vi "CarSimulator.vi"(10 "Steering Control":dbl, 11 "Brake/Gas Control":dbl) -> (1 "Acceleration":dbl, 2 "Velocity":dbl, 3 "Position":dbl)   [LabVIEW 2020]
panel:
  in  "Gas to Acceleration Scalar":dbl=1.8
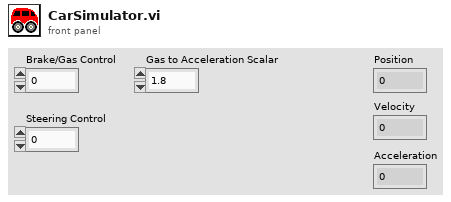
[diagram p1: front panel]
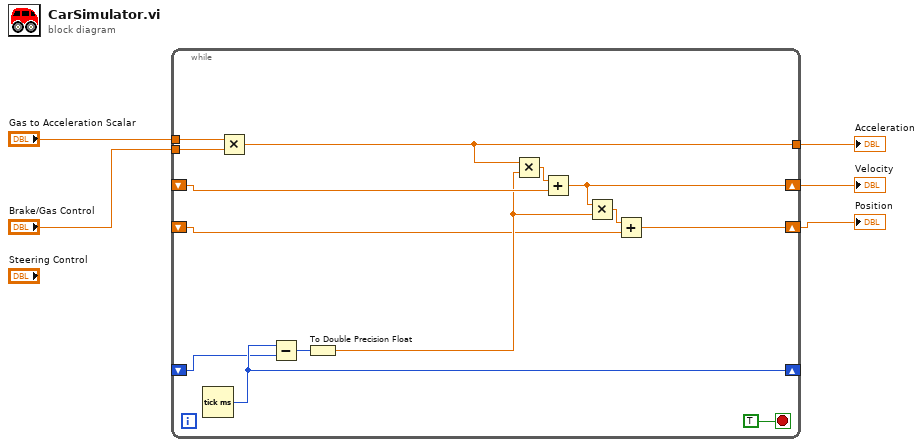
[diagram p0: block diagram]
diagram:
  n1 = while {
    shift-right: [w7] -> _
    shift-left: _ -> [w6]
    tunnel: "Gas to Acceleration Scalar" -> [w18]
    tunnel: "Brake/Gas Control" -> [w17]
    tunnel: [w15] -> w3
    shift-right: [w11] -> w2
    shift-left: _ -> [w16]
    shift-right: [w9] -> w1
    shift-left: _ -> [w8]
    stop <- TRUE stop-if-true
    n2 = Tick Count (ms)() -> (millisecond timer value=w7:u32)
    n3 = Multiply(x=w18, y=w17) -> (x*y=w15:dbl)
    n4 = Subtract(x=w7, y=w6) -> (x-y=w13:u32)
    n5 = To Double Precision Float(number=w13) -> (double precision float=w10:dbl)
    n6 = Multiply(x=w15, y=w10) -> (x*y=w14:dbl)
    n7 = Add(x=w14, y=w16) -> (x+y=w11:dbl)
    n8 = Multiply(x=w11, y=w10) -> (x*y=w12:dbl)
    n9 = Add(x=w12, y=w8) -> (x+y=w9:dbl)
  }
  "Position" <- w1
  "Velocity" <- w2
  "Acceleration" <- w3
